vi "Make VI Standard.vi"(6 "Label.Font:Bold (T)":bool=TRUE, 7 "Auto Error Handling (F)":bool, 8 "error in":errorcluster, 9 "Label.FontColor":u32(colorbox), 10 "Label.BGColor":u32(colorbox)=16777216, 11 "vi path":path=path "C:/ATS Development/Code/Test Cases/Test Case, Waveform Attributes.vi") -> (0 "error out":errorcluster, 2 "Label Count":i32=7)   [LabVIEW 2010]
panel:
  out "Auto Error Handling":bool
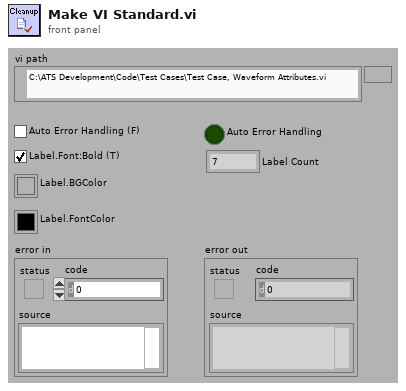
[diagram p1: front panel]
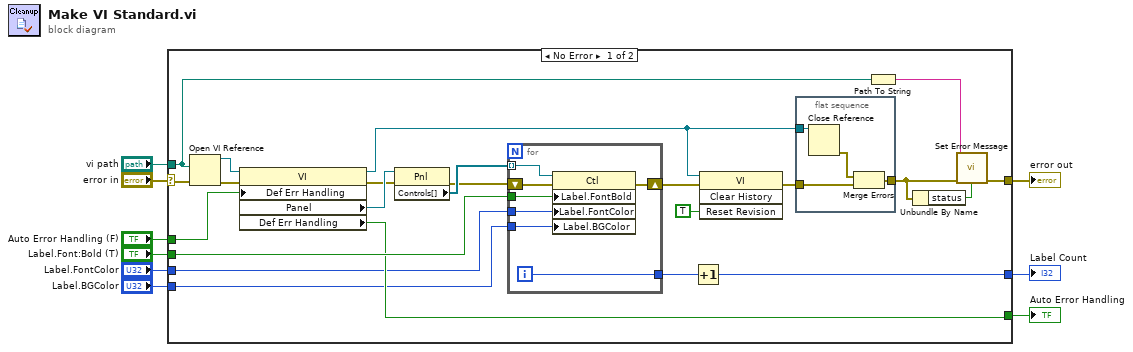
[diagram p0: block diagram]
diagram:
  n1 = case shown="No Error" "error in" {
    selector: "error in" -> [w16 w44]
    tunnel: "Label.Font:Bold (T)" -> [w28 _]
    tunnel: [w24 _] -> w8
    tunnel: [w23 _] -> w7
    tunnel: "Label.FontColor" -> [w22 _]
    tunnel: "Label.BGColor" -> [w21 _]
    tunnel: "Auto Error Handling (F)" -> [w20 _]
    tunnel: [w19 w44] -> w3
    tunnel: "vi path" -> [w17 _]
    frame No Error {
      n2 = Open VI Reference(vi path=w17, error in (no error)=w16) -> (vi reference=w27:refnum<vi>, error out=w26:errorcluster)  [unwired: 4 in]
      n3 = property class="VI"(reference=w27, error in=w26, "Def Err Handling"=w20) -> (reference out=w11:refnum<vi>, error out=w30:errorcluster, "Panel"=w31:refnum<vi>, "Def Err Handling"=w24:bool)
      n4 = property class="Pnl"(reference=w31, error in=w30) -> (error out=w29:errorcluster, "Controls[]"=w32:refnum<vi>[])  [unwired: 1 out]
      n5 = for {
        tunnel: w32 -> [w43] mode=indexing
        shift-right: [w41] -> w13
        shift-left: w29 -> [w42]
        tunnel: w28 -> [w40]
        tunnel: [w39] -> w25
        tunnel: w22 -> [w38]
        tunnel: w21 -> [w37]
        i -> [w39]
        n6 = property class="Ctl"(reference=w43, error in=w42, "Label.FontBold"=w40, "Label.FontColor"=w38, "Label.BGColor"=w37) -> (error out=w41:errorcluster)  [unwired: 1 out]
      }
      n7 = Increment(x=w25) -> (x+1=w23:i32)
      n8 = invoke class="VI" method="Clear History"(reference=w11, error in=w13, "Reset Revision"=TRUE) -> (error out=w12:errorcluster)  [unwired: 1 in, 3 out]
      n9 = flat-sequence {
        tunnel: w11 -> [w36]
        tunnel: [w34] -> w15
        tunnel: w12 -> [w33]
        frame #0 {
          n10 = Close Reference(reference=w36) -> (error out=w35:errorcluster)  [unwired: 1 in]
          n11 = Merge Errors(w35, w33) -> (w34:errorcluster)
        }
      }
      n12 = Path To String(path=w17) -> (string=w18:string)
      n13 = Unbundle By Name(w15) -> ("status"=w14:bool)
      n14 = call "Set Error Message.vi"("Enable (T)"=w14, "error in"=w15, "Message"=w18) -> ("error out"=w19:errorcluster)  [unwired: 5 in]
    }
    frame Error {
    }
  }
  "Auto Error Handling" <- w8
  "error out" <- w3
  "Label Count" <- w7
